vi "Check_Particle_State_NextTime_ver2.vi"(0 "Particle State at T":T3(array[cluster]), 1 "Torque?":bool, 2 "Torque":dbl, 3 "Rot diffusion\nfor Cargo?":bool, 5 "Tau_On":i32, 7 "Tau_Off":i32, 11 "Center State at T":T1, 12 "Asymmetry (X, Y)":dbl[](array[numeric]), 13 "SD":dbl, 14 "Rot diffusion\nfor Cargo":dbl format="%#_13g") -> (4 "Particle State at T+1":T2(array[cluster]), 15 "New Center State at T":T1)   [LabVIEW 2020]
uses:
  <vilib>/gmath/statdist.llb/Normal Random.vi
  <vilib>/gmath/NI_Gmath.lvlib
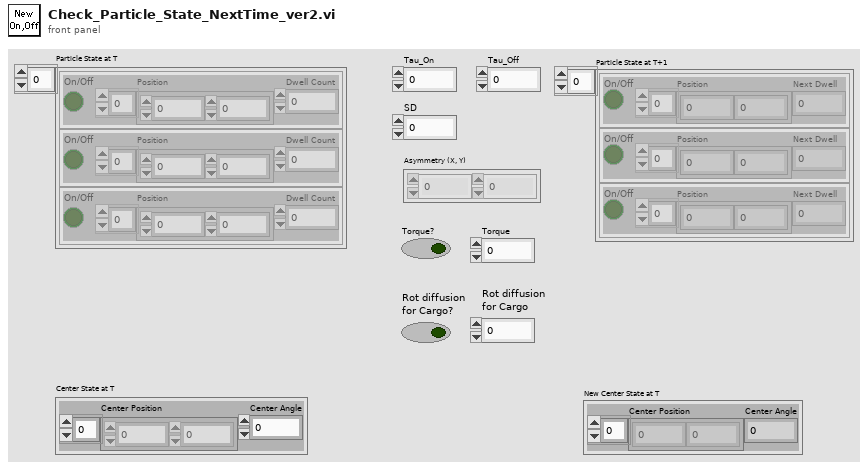
[diagram p1: front panel]
types:
  T1 = cluster{"Center Position":dbl[], "Center Angle":dbl}
  T2 = cluster{"On/Off":bool, "Position":dbl[], "Next Dwell":i32}[]
  T3 = cluster{"On/Off":bool, "Position":dbl[], "Dwell Count":i32}[]
  T4 = cluster{"On/Off":bool, "Position":dbl[], "Next Dwell":i32}
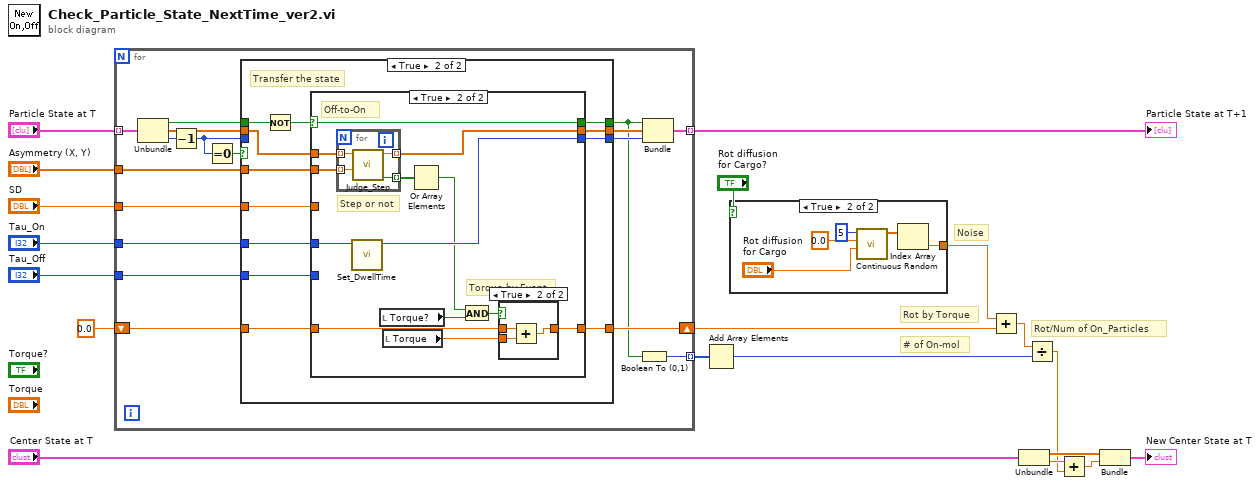
[diagram p0: block diagram]
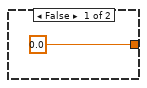
[diagram p2: hidden frame]
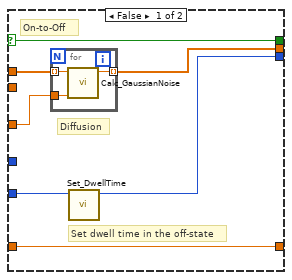
[diagram p4: hidden frame]
diagram:
  # "# of On-mol"
  # "Rot by Torque"
  # "Noise"
  # "Rot/Num of On_Particles"
  n1 = for {
    tunnel: "Particle State at T" -> [w36] mode=indexing
    tunnel: "Tau_On" -> [w30]
    tunnel: "Tau_Off" -> [w28]
    tunnel: [w27] -> w16 mode=indexing
    tunnel: "Asymmetry (X, Y)" -> [w25]
    tunnel: "SD" -> [w24]
    shift-right: [w22] -> w3
    shift-left: 0.0 -> [w23]
    tunnel: [w20] -> w12 mode=indexing
    n2 = Unbundle(w36) -> ("On/Off"=w33:bool, "Position"=w32:dbl[], "Dwell Count"=w35:i32)
    n3 = Decrement(x=w35) -> (x-1=w26:i32)
    n4 = Equal To 0?(x=w26) -> (x = 0?=w34:bool)
    n5 = case shown="TRUE" w34 {
      tunnel: w33 -> [w40 w48]
      tunnel: [w40 w44] -> w21
      tunnel: w32 -> [w39 w47]
      tunnel: [w39 w45] -> w31
      tunnel: w30 -> [_ w52]
      tunnel: [w38 w51] -> w29
      tunnel: w28 -> [_ w50]
      tunnel: w26 -> [w38 _]
      tunnel: w25 -> [_ w46]
      tunnel: w24 -> [_ w43]
      tunnel: w23 -> [w37 w41]
      tunnel: [w37 w42] -> w22
      frame False {
        # "Not transfering state"
      }
      frame True {
        # "Transfer the state"
        n6 = Not(x=w48) -> (.not. x?=w49:bool)
        n7 = case shown="TRUE" w49 {
          selector: w49 -> [w57 w66]
          tunnel: w52 -> [_ w75]
          tunnel: [w58 w74] -> w51
          tunnel: w50 -> [w59 _]
          tunnel: w47 -> [w56 w73]
          tunnel: w46 -> [_ w72]
          tunnel: [w55 w70] -> w45
          tunnel: [w57 w66] -> w44
          tunnel: w43 -> [w54 _]
          tunnel: w41 -> [w53 w69]
          tunnel: [w53 w71] -> w42
          frame False {
            # "On-to-Off"
            # "Set dwell time in the off-state"
            # "Diffusion"
            n8 = for {
              tunnel: w56 -> [w62] mode=indexing
              tunnel: [w61] -> w55 mode=indexing
              tunnel: w54 -> [w60]
              n9 = call "Calc_GaussianNoise.vi"("SD"=w60, "Start Position"=w62) -> ("Final Position"=w61:dbl)  [unwired: 9 in]
            }
            n10 = call "Set_DwellTime.vi"("Tau"=w59) -> ("Next Dwell"=w58:i32)  [unwired: 10 in]
          }
          frame True {
            # "Off-to-On"
            # "Step or not"
            # "Torque by Event"
            n11 = for {
              tunnel: w73 -> [w83] mode=indexing
              tunnel: w72 -> [w82] mode=indexing
              tunnel: [w81] -> w70 mode=indexing
              tunnel: [w80] -> w64 mode=indexing
              n12 = call "Judge_Step.vi"("Asymmetry"=w82, "Position"=w83) -> ("Off To On?"=w80:bool, "New Position"=w81:dbl)  [unwired: 8 in]
            }
            n13 = call "Set_DwellTime.vi"("Tau"=w75) -> ("Next Dwell"=w74:i32)  [unwired: 10 in]
            n14 = local read "Torque?"() -> (w68:bool)
            n15 = local read "Torque"() -> (w65:dbl)
            n16 = Or Array Elements(Boolean array=w64) -> (logical OR=w63:bool)
            n17 = And(x=w63, y=w68) -> (x .and. y?=w67:bool)
            n18 = case shown="TRUE" w67 {
              tunnel: w69 -> [w76 w78]
              tunnel: [w76 w77] -> w71
              tunnel: w65 -> [_ w79]
              frame False {
              }
              frame True {
                n19 = Add(x=w78, y=w79) -> (x+y=w77:dbl)
              }
            }
          }
        }
      }
    }
    n20 = Boolean To (0,1)(Boolean=w21) -> (0, 1=w20:i16)
    n21 = Bundle("On/Off"=w21, "Position"=w31, "Next Dwell"=w29) -> (w27:T4)  [unwired: 1 in]
  }
  "Particle State at T+1" <- w16
  n22 = Add Array Elements(numeric array=w12) -> (sum=w5:i16)
  n23 = case shown="TRUE" "Rot diffusion\nfor Cargo?" {
    tunnel: [0.0 w86] -> w2
    frame False {
    }
    frame True {
      n24 = call-poly <vilib>:"Continuous Random.vi"("std"="Rot diffusion\nfor Cargo", "mean"=0.0, "samples"=5) -> ("normal random data"=w89:dbl[])  [unwired: 7 in, 1 out]
      n25 = Index Array(array=w89) -> (element=w86:dbl)  [unwired: 1 in]
    }
  }
  n26 = Add(x=w2, y=w3) -> (x+y=w1:dbl)
  n27 = Unbundle("Center State at T") -> ("Center Position"=w10:dbl[], "Center Angle"=w9:dbl)
  n28 = Divide(x=w1, y=w5) -> (x/y=w8:dbl)
  n29 = Add(x=w9, y=w8) -> (x+y=w7:dbl)
  n30 = Bundle("Center Position"=w10, w7) -> (→"New Center State at T":cluster{"Center Position":dbl[], dbl})  [unwired: 1 in]
